vi "TDMS Append Run to File.vi"(7 "TDMS Path to Append":path, 8 "error in (no error)":errorcluster, 10 "TDMS Path":path, 11 "TDMS File to Append Ref":refnum<k34>) -> (0 "error out":errorcluster, 3 "TDMS Path":path)   [LabVIEW 2011]
uses:
  Summitek EXT/OpenG EXT/array/array.llb/Remove Duplicates from 1D Array (DBL)__ogtk.vi
  Summitek EXT/OpenG EXT/array/array.llb/Delete Elements from 1D Array (String)__ogtk.vi
  Summitek EXT/OpenG EXT/array/array.llb/Delete Elements from 1D Array (DBL)__ogtk.vi
  server lib/Spartan Version.vi
  Summitek EXT/OpenG EXT/file/file.llb/Convert File Extension (Path)__ogtk.vi
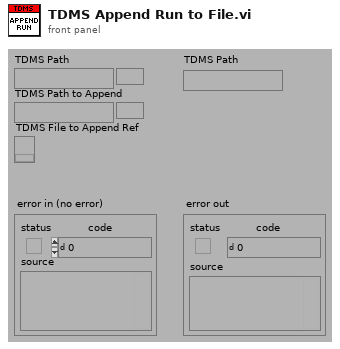
[diagram p1: front panel]
types:
  T1 = enum16{"open", "open or create", "create or replace", "create", "open (read-only)"}
  T2 = typedef "OGAB Version.ctl" = cluster{"Version":string, "Build Number":u32, "Build Date/Time":dbl}
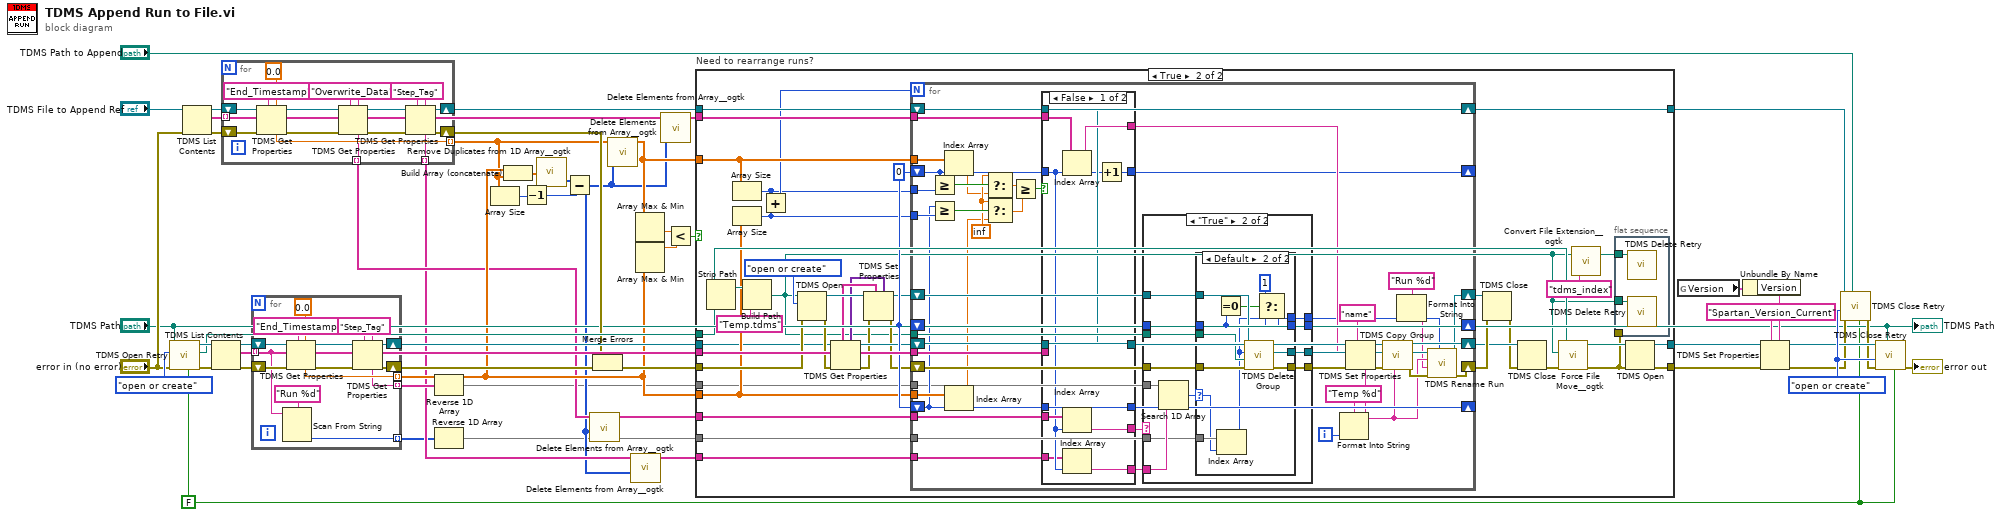
[diagram p0: block diagram]
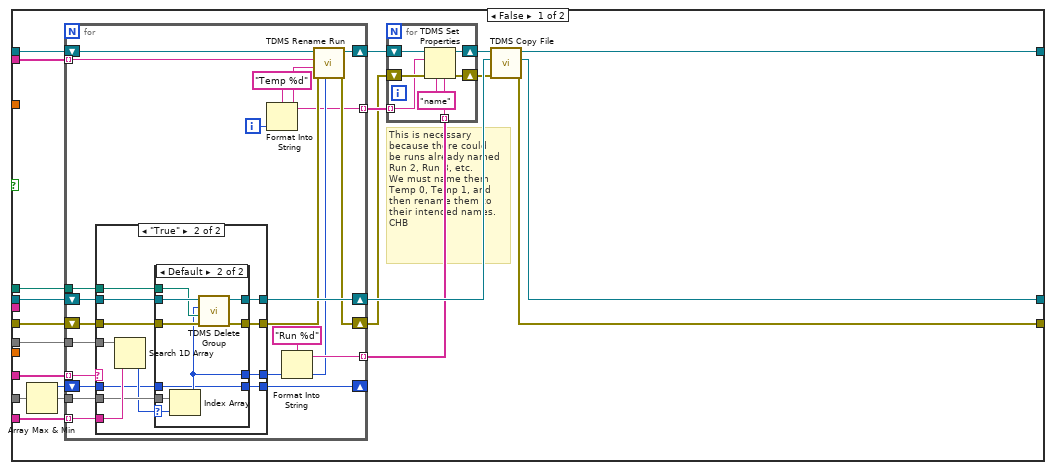
[diagram p2: hidden frame]
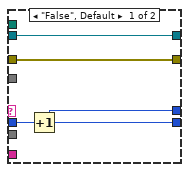
[diagram p3: hidden frame]
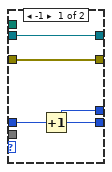
[diagram p4: hidden frame]
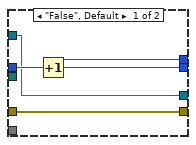
[diagram p5: hidden frame]
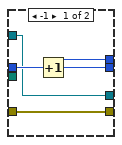
[diagram p6: hidden frame]
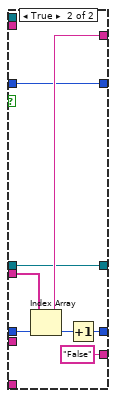
[diagram p7: hidden frame]
diagram:
  w19 = FALSE ("Exclusive Access? (T)")
  w38 = T1."open or create" ("operation (0:open)")
  n1 = call "TDMS Open Retry.vi"("Lock File? (T)"=w19, "error in (no error)"="error in (no error)", "Operation (0:open)"=T1."open or create" ("operation (0:open)"), "Path"="TDMS Path") -> ("error out"=w51:errorcluster, "TDMS Temp Path"=w28:path, "TDMS File Ref"=w50:refnum<k34>)  [unwired: 1 in, 4 out]
  n2 = TDMS List Contents(4:"error in (no error)", 7:"TDMS File to Append Ref") -> (0:w48:errorcluster, 2:w17:string[], 3:w47:refnum<k34>)  [unwired: 2 out]
  n3 = TDMS List Contents(4:w51, 7:w50) -> (0:w45:errorcluster, 2:w27:string[], 3:w46:refnum<k34>)  [unwired: 2 out]
  n4 = for {
    tunnel: w17 -> [w67] mode=indexing
    shift-right: [w53] -> w25
    shift-left: w48 -> [w68]
    shift-right: [w54] -> w42
    shift-left: w47 -> [w69]
    tunnel: [w65] -> w10 mode=indexing
    tunnel: [w61] -> w9 mode=indexing
    tunnel: [w52] -> w5 mode=indexing
    w58 = "Step_Tag" ("property name")
    w62 = "Overwrite_Data" ("property name")
    n5 = TDMS Get Properties(5:0.0 ("default (0 I32)"), 7:"End_Timestamp" ("property name"), 8:w68, 10:w67, 11:w69) -> (0:w63:errorcluster, 2:w60:string, 3:w64:refnum<k34>, 4:w65:dbl)  [unwired: 1 in, 2 out]
    n6 = TDMS Get Properties(5:w62, 7:w62, 8:w63, 10:w60, 11:w64) -> (0:w57:errorcluster, 2:w55:string, 3:w56:refnum<k34>, 4:w61:string)  [unwired: 1 in, 2 out]
    n7 = TDMS Get Properties(5:w58, 7:w58, 8:w57, 10:w55, 11:w56) -> (0:w53:errorcluster, 3:w54:refnum<k34>, 4:w52:string)  [unwired: 1 in, 3 out]
  }
  n8 = for {
    tunnel: w27 -> [w79] mode=indexing
    shift-right: [w74] -> w26
    shift-left: w45 -> [w83]
    shift-right: [w73] -> w41
    shift-left: w46 -> [w84]
    tunnel: [w81] -> w14 mode=indexing
    tunnel: [w78] -> w1 mode=indexing
    tunnel: [w71] -> w8 mode=indexing
    w72 = "Step_Tag" ("property name")
    n9 = Scan From String(format string="Run %d", input string=w79) -> (output 1=w78:i32)  [unwired: 2 in, 4 out]
    n10 = TDMS Get Properties(5:0.0 ("default (0 I32)"), 7:"End_Timestamp" ("property name"), 8:w83, 10:w79, 11:w84) -> (0:w75:errorcluster, 2:w70:string, 3:w76:refnum<k34>, 4:w81:dbl)  [unwired: 1 in, 2 out]
    n11 = TDMS Get Properties(5:w72, 7:w72, 8:w75, 10:w70, 11:w76) -> (0:w74:errorcluster, 3:w73:refnum<k34>, 4:w71:string)  [unwired: 1 in, 3 out]
  }
  n12 = Reverse 1D Array(array=w8) -> (reversed array=w3:string[])
  n13 = Reverse 1D Array(array=w1) -> (reversed array=w2:i32[])
  n14 = Array Size(array=w10) -> (size(s)=w13:i32)
  n15 = Build Array (concatenate)(w14, w10) -> (w18:dbl[])
  n16 = Decrement(x=w13) -> (x-1=w12:i32)
  n17 = call-poly "Remove Duplicates from 1D Array__ogtk.vi"("Input Array"=w18) -> ("indices of removed elements"=w11:i32[])  [unwired: 1 out]
  n18 = Subtract(x=w11, y=w12) -> (x-y=w4:i32[])
  n19 = call-poly "Delete Elements from Array__ogtk.vi"("indices"=w4, "array"=w9) -> ("array w/ subset deleted"=w7:string[])  [unwired: 8 in, 1 out]
  n20 = Merge Errors(w25, w26) -> (w24:errorcluster)
  n21 = call-poly "Delete Elements from Array__ogtk.vi"("indices"=w4, "array"=w10) -> ("array w/ subset deleted"=w15:dbl[])  [unwired: 8 in, 1 out]
  n22 = call-poly "Delete Elements from Array__ogtk.vi"("indices"=w4, "array"=w5) -> ("array w/ subset deleted"=w6:string[])  [unwired: 8 in, 1 out]
  n23 = Array Max & Min(array=w15) -> (min value=w40:dbl)  [unwired: 3 out]
  n24 = Array Max & Min(array=w14) -> (max value=w44:dbl)  [unwired: 3 out]
  n25 = call-poly "Delete Elements from Array__ogtk.vi"("indices"=w4, "array"=w17) -> ("array w/ subset deleted"=w16:string[])  [unwired: 8 in, 1 out]
  n26 = Less?(x=w40, y=w44) -> (x < y?=w43:bool)
  n27 = case "Need to rearrange runs?" shown="True" w43 {
    tunnel: w42 -> [w104 w201]
    tunnel: w41 -> [w99 w174]
    tunnel: w16 -> [w103 w195]
    tunnel: [w102 w200] -> w39
    tunnel: [w101 w186] -> w33
    tunnel: [w89 w188] -> w34
    tunnel: w28 -> [w100 w189]
    tunnel: w7 -> [w98 w193]
    tunnel: w14 -> [_ w181]
    tunnel: w15 -> [_ w182]
    tunnel: w27 -> [_ w194]
    tunnel: w24 -> [w91 w185]
    tunnel: w2 -> [w85 w162]
    tunnel: w3 -> [w86 w164]
    tunnel: w6 -> [w87 w163]
    frame False {
      # "This is necessary\nbecause there could\nbe runs already named\nRun 2, Run 3, etc.\nWe must name them\nTemp 0, Temp 1, and\nthen rename them to\ntheir intended names.\nCHB"
      n28 = Array Max & Min(array=w85) -> (max value=w88:i32)  [unwired: 3 out]
      n29 = for {
        shift-right: [w119] -> w96
        shift-left: w104 -> [w120]
        tunnel: w103 -> [w118] mode=indexing
        shift-right: [w112] -> _
        shift-left: w88 -> [w127]
        tunnel: w100 -> [w131]
        shift-right: [w121] -> w90
        shift-left: w91 -> [w129]
        tunnel: w98 -> [w128] mode=indexing
        shift-right: [w126] -> w97
        shift-left: w99 -> [w130]
        tunnel: [w124] -> w93 mode=indexing
        tunnel: [w116] -> w92 mode=indexing
        tunnel: w87 -> [w115] mode=indexing
        tunnel: w86 -> [w114]
        tunnel: w85 -> [w113]
        i -> [w123]
        n30 = case shown="\"True\"" w128 {
          tunnel: w130 -> [w135 w148]
          tunnel: w129 -> [w136 w147]
          tunnel: [w136 w146] -> w122
          tunnel: [w135 w145] -> w126
          tunnel: w131 -> [_ w144]
          tunnel: w127 -> [w134 w138]
          tunnel: [w133 w139] -> w117
          tunnel: w115 -> [_ w142]
          tunnel: w114 -> [_ w143]
          tunnel: w113 -> [_ w141]
          tunnel: [w133 w137] -> w112
          frame "False", Default {
            n31 = Increment(x=w134) -> (x+1=w133:i32)
          }
          frame "True" {
            n32 = Search 1D Array(1D array=w143, element=w142) -> (index of element=w140:i32)  [unwired: 1 in]
            n33 = case shown="Default" w140 {
              selector: w140 -> [_ w155]
              tunnel: w148 -> [w151 w161]
              tunnel: w147 -> [w152 w160]
              tunnel: [w152 w159] -> w146
              tunnel: [w151 w158] -> w145
              tunnel: w144 -> [_ w157]
              tunnel: w141 -> [_ w156]
              tunnel: [w149 w154] -> w139
              tunnel: w138 -> [w150 w153]
              tunnel: [w149 w153] -> w137
              frame -1 {
                n34 = Increment(x=w150) -> (x+1=w149:i32)
              }
              frame Default {
                n35 = Index Array(array=w156, index=w155) -> (element=w154:i32)
                n36 = call "TDMS Delete Group.vi"("error in (no error)"=w160, "File Path In"=w157, "Run to Delete"=w154, "TDMS File Ref"=w161) -> ("error out"=w159:errorcluster, "TDMS File Ref"=w158:refnum<k34>)  [unwired: 2 in, 4 out]
              }
            }
          }
        }
        n37 = Format Into String(format string="Temp %d", w123) -> (resulting string=w116:string)  [unwired: 2 in, 1 out]
        n38 = Format Into String(format string="Run %d", w117) -> (resulting string=w124:string)  [unwired: 2 in, 1 out]
        n39 = call "TDMS Rename Run.vi"("Run Number"=w117, "error in (no error)"=w122, "Run Name (\"\")"=w116, "Run to Rename (\"\")"=w118, "TDMS File Ref In"=w120) -> ("error out"=w121:errorcluster, "TDMS File Ref Out"=w119:refnum<k34>)  [unwired: 5 in]
      }
      n40 = for {
        shift-right: [w108] -> w95
        shift-left: w90 -> [w109]
        shift-right: [w107] -> w94
        shift-left: w96 -> [w110]
        tunnel: w93 -> [w106] mode=indexing
        tunnel: w92 -> [w105] mode=indexing
        n41 = TDMS Set Properties(5:w106, 7:"name" ("Property Name"), 8:w109, 10:w105, 11:w110) -> (0:w108:errorcluster, 3:w107:refnum<k34>)  [unwired: 1 in, 2 out]
      }
      n42 = call "TDMS Copy File.vi"("error in"=w95, "tdms dest in"=w97, "tdms source in"=w94) -> ("error out"=w89:errorcluster, "tdms dest out"=w101:refnum<k34>, "tdms source out"=w102:refnum<k34>)  [unwired: 6 in]
    }
    frame True {
      w184 = 0 ("default (0 I32)")
      n43 = Strip Path(path=w189) -> (stripped path=w198:path)  [unwired: 1 out]
      n44 = Array Size(array=w182) -> (size(s)=w179:i32)
      n45 = Array Size(array=w181) -> (size(s)=w178:i32)
      n46 = Build Path(base path=w198, name or relative path="Temp.tdms" ("property name")) -> (appended path=w165:path)
      n47 = Add(x=w179, y=w178) -> (x+y=w180:i32)
      n48 = TDMS Open(8:w185, 10:T1."open or create" ("operation (0:open)"), 11:w165) -> (0:w175:errorcluster, 3:w177:refnum<k34>)  [unwired: 3 in]
      n49 = TDMS Get Properties(8:w175, 11:w174) -> (0:w172:errorcluster, 3:w173:refnum<k34>, 4:w169:variant[], 6:w170:string[])  [unwired: 4 in, 2 out]
      n50 = TDMS Set Properties(5:w169, 7:w170, 8:w172, 11:w177) -> (0:w171:errorcluster, 3:w176:refnum<k34>)  [unwired: 2 in, 2 out]
      n51 = for {
        N: w180 -> [_]
        tunnel: w182 -> [w232]
        tunnel: w181 -> [w230]
        shift-right: [w215] -> w192
        shift-left: w171 -> [w246]
        shift-right: [w233] -> w191
        shift-left: w173 -> [w233]
        shift-right: [w234] -> w200
        shift-left: w201 -> [w234]
        shift-right: [w231] -> _
        shift-left: w184 -> [w227]
        shift-right: [w247] -> _
        shift-left: w184 -> [w224]
        shift-right: [w216] -> w196
        shift-left: w176 -> [w242]
        tunnel: w193 -> [w248]
        shift-right: [w204] -> _
        shift-left: w184 -> [w245]
        tunnel: w165 -> [w244]
        tunnel: w194 -> [w249]
        tunnel: w195 -> [w250]
        tunnel: w179 -> [w226]
        tunnel: w178 -> [w225]
        tunnel: w164 -> [w208]
        tunnel: w163 -> [w207]
        tunnel: w162 -> [w205]
        i -> [w228]
        w221 = inf
        n52 = Greater Or Equal?(x=w227, y=w226) -> (x >= y?=w223:bool)
        n53 = Greater Or Equal?(x=w224, y=w225) -> (x >= y?=w222:bool)
        n54 = Index Array(array=w232, index=w227) -> (element=w220:dbl)
        n55 = Index Array(array=w230, index=w224) -> (element=w218:dbl)
        n56 = Select(t=w221, s=w223, f=w220) -> (s? t:f=w219:dbl)
        n57 = Select(t=w221, s=w222, f=w218) -> (s? t:f=w217:dbl)
        n58 = Greater Or Equal?(x=w219, y=w217) -> (x >= y?=w251:bool)
        n59 = case shown="False" w251 {
          tunnel: w234 -> [w291 _]
          tunnel: w233 -> [_ w298]
          tunnel: w250 -> [w293 _]
          tunnel: w249 -> [_ w299]
          tunnel: w248 -> [w287 _]
          tunnel: w224 -> [w289 w297]
          tunnel: w227 -> [w286 w295]
          tunnel: [w291 w298] -> w239
          tunnel: [w292 w300] -> w237
          tunnel: [w289 w296] -> w247
          tunnel: [w290 w295] -> w231
          tunnel: [w288 "False" ("property name")] -> w243
          tunnel: w207 -> [w285 _]
          tunnel: [w284 _] -> w206
          frame False {
            n60 = Index Array(array=w293, index=w286) -> (element=w292:string)
            n61 = Index Array(array=w287, index=w286) -> (element=w288:string)
            n62 = Index Array(array=w285, index=w286) -> (element=w284:string)
            n63 = Increment(x=w286) -> (x+1=w290:i32)
          }
          frame True {
            n64 = Index Array(array=w299, index=w297) -> (element=w300:string)
            n65 = Increment(x=w297) -> (x+1=w296:i32)
          }
        }
        n66 = case shown="\"True\"" w243 {
          tunnel: w246 -> [w255 w267]
          tunnel: [w255 w266] -> w240
          tunnel: w244 -> [_ w265]
          tunnel: w245 -> [w254 w262]
          tunnel: [w252 w261] -> w210
          tunnel: w242 -> [w253 w263]
          tunnel: [w253 w264] -> w241
          tunnel: w208 -> [_ w260]
          tunnel: w206 -> [_ w259]
          tunnel: w205 -> [_ w257]
          tunnel: [w252 w256] -> w204
          frame "False", Default {
            n67 = Increment(x=w254) -> (x+1=w252:i32)
          }
          frame "True" {
            n68 = Search 1D Array(1D array=w260, element=w259) -> (index of element=w258:i32)  [unwired: 1 in]
            n69 = case shown="Default" w258 {
              selector: w258 -> [_ w275]
              tunnel: w267 -> [w270 w283]
              tunnel: [w270 w282] -> w266
              tunnel: w265 -> [_ w281]
              tunnel: [w269 w280] -> w264
              tunnel: w263 -> [w269 w279]
              tunnel: w262 -> [w271 w274]
              tunnel: [w268 w272] -> w261
              tunnel: w257 -> [_ w276]
              tunnel: [w268 w273] -> w256
              frame -1 {
                n70 = Increment(x=w271) -> (x+1=w268:i32)
              }
              frame Default {
                n71 = Equal To 0?(x=w274) -> (x = 0?=w278:bool)
                n72 = Index Array(array=w276, index=w275) -> (element=w272:i32)
                n73 = call "TDMS Delete Group.vi"("error in (no error)"=w283, "File Path In"=w281, "Run to Delete"=w272, "TDMS File Ref"=w279) -> ("error out"=w282:errorcluster, "TDMS File Ref"=w280:refnum<k34>)  [unwired: 2 in, 4 out]
                n74 = Select(t=1 ("default (0 I32)"), s=w278, f=w274) -> (s? t:f=w273:i32)
              }
            }
          }
        }
        n75 = Format Into String(format string="Temp %d", w228) -> (resulting string=w212:string)  [unwired: 2 in, 1 out]
        n76 = TDMS Set Properties(5:w212, 7:"name" ("Property Name"), 8:w240, 10:w237, 11:w239) -> (0:w236:errorcluster, 3:w235:refnum<k34>)  [unwired: 1 in, 2 out]
        n77 = call "TDMS Copy Group.vi"("group name"=w212, "error in"=w236, "tdms dest in"=w241, "tdms source in"=w235) -> ("error out"=w213:errorcluster, "tdms dest out"=w214:refnum<k34>)  [unwired: 5 in, 1 out]
        n78 = Format Into String(format string="Run %d", w210) -> (resulting string=w209:string)  [unwired: 2 in, 1 out]
        n79 = call "TDMS Rename Run.vi"("Run Number"=w210, "error in (no error)"=w213, "Run Name (\"\")"=w209, "Run to Rename (\"\")"=w212, "TDMS File Ref In"=w214) -> ("error out"=w215:errorcluster, "TDMS File Ref Out"=w216:refnum<k34>)  [unwired: 5 in]
      }
      n80 = TDMS Close(8:w192, 11:w196) -> (0:w190:errorcluster)  [unwired: 1 out]
      n81 = TDMS Close(8:w190, 11:w191) -> (0:w167:errorcluster)  [unwired: 1 out]
      n82 = call "Force File Move__ogtk.vi"("error in (no error)"=w167, "source"=w165, "target"=w189) -> ("error out"=w168:errorcluster, "target out"=w187:path)  [unwired: 3 in]
      n83 = call-poly "Convert File Extension__ogtk.vi"("new ending (none)"="tdms_index" ("property name"), "file name"=w165) -> ("new filename"=w166:path)  [unwired: 1 out]
      n84 = flat-sequence {
        tunnel: w168 -> [_]
        tunnel: w166 -> [w203]
        tunnel: w165 -> [w202]
        frame #0 {
          n85 = call "TDMS Delete Retry.vi"("path (use dialog)"=w203) -> ()  [unwired: 11 out]
          n86 = call "TDMS Delete Retry.vi"("path (use dialog)"=w202) -> ()  [unwired: 11 out]
        }
      }
      n87 = TDMS Open(8:w168, 11:w187) -> (0:w188:errorcluster, 3:w186:refnum<k34>)  [unwired: 4 in]
    }
  }
  n88 = global read "Spartan Version.vi" "Version"() -> (w36:T2)
  n89 = Unbundle By Name(w36) -> ("Version"=w35:string)
  n90 = TDMS Set Properties(5:w35, 7:"Spartan_Version_Current" ("property name"), 8:w34, 11:w33) -> (0:w23:errorcluster, 3:w32:refnum<k34>)  [unwired: 2 in, 2 out]
  n91 = call "TDMS Close Retry.vi"("Release File? (T)"=w19, "TDMS Path"="TDMS Path to Append", "error in (no error)"=w23, "Operation (0:open)"=w38, "TDMS File Ref"=w39) -> ("error out"=w22:errorcluster)  [unwired: 6 out]
  n92 = call "TDMS Close Retry.vi"("Release File? (T)"=w19, "TDMS Path"="TDMS Path", "error in (no error)"=w22, "Operation (0:open)"=w38, "TDMS File Ref"=w32) -> ("error out"=→"error out":errorcluster)  [unwired: 6 out]
  "TDMS Path" <- "TDMS Path"
